vi "SystemExecTest.vi"() -> ()   [LabVIEW 2025]
panel:
  in  "path":path
  in  "standard input":string
  out "error out":errorcluster
  out "standard output":string
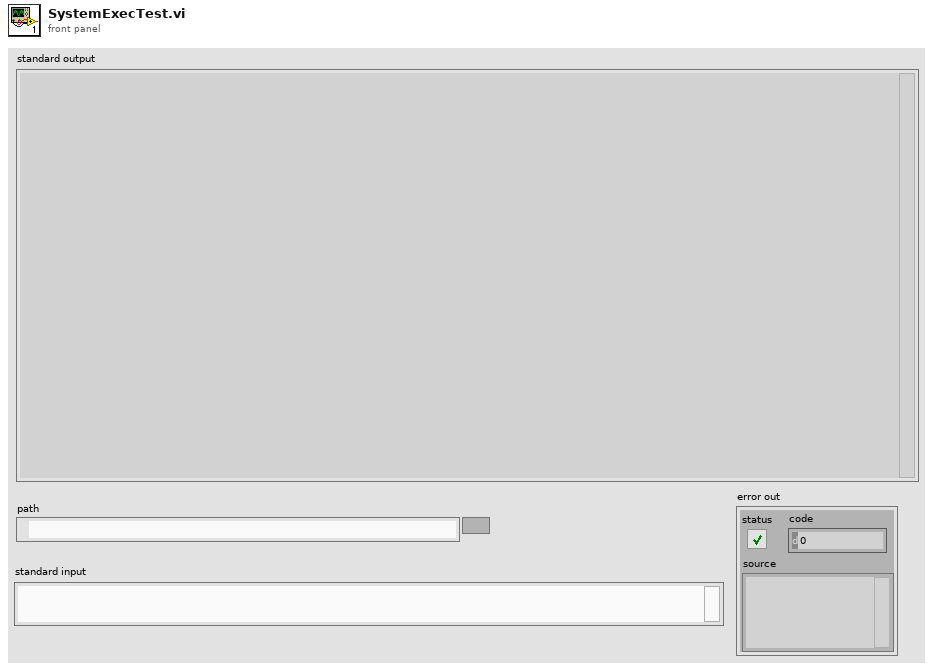
[diagram p1: front panel]
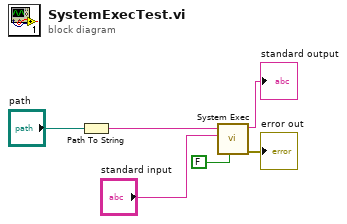
[diagram p0: block diagram]
diagram:
  n1 = Path To String(path="path") -> (string=w2:string)
  n2 = call <vilib>:"System Exec.vi"("run minimized? (F)"=FALSE, "standard input"="standard input", "command line"=w2) -> ("error out"=→"error out":errorcluster, "standard output"=→"standard output":string)  [unwired: 5 in, 2 out]
